vi "Dash_Hopper_Testing.vi"() -> ()   [LabVIEW 2017, in "Hopper System.lvlib"]
uses:
  Hopper System.lvlib
  Cluster_CMD to SM Data.ctl
  ENUM_Firing_State.ctl
  _SHARE ALL/Global Share All/Global_STOP.vi
  Globals/Global_CMD to SM Data.vi
  Global_Line-Fake.vi
  Global_SM_Data Out.vi
panel:
  in  "Line Sensor-Fake_Testor":bool
  in  "Hopper Stop_CMD":bool
  out "Hopper_SM_Loader Speed":dbl
  out "Hopper_SM_Center Speed":dbl
  in  "Inner Motor Speed":dbl=0.4
  in  "STOP":bool
  in  "Loader Speed":dbl=0.4
  in  "Hopper_CMD":T1={"Enable Loading"=FALSE, "Disable Loading"=FALSE, "Fireing State"=enum."No Fireing", "Time Limit Loading"=5.0, "Time Limit Rapid"=2.0, "Rapid Fire Shot Limit"=0, "Shotgun Fire Shot Limit"=0}
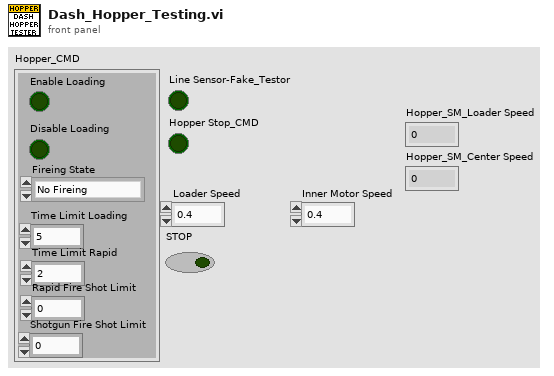
[diagram p1: front panel]
types:
  T1 = typedef "Hopper System.lvlib/Cluster_CMD to SM Data.ctl" = cluster{"Enable Loading":bool, "Disable Loading":bool, "Fireing State":T2, "Time Limit Loading":dbl, "Time Limit Rapid":dbl, "Rapid Fire Shot Limit":i32, "Shotgun Fire Shot Limit":i32}
  T2 = typedef "Hopper System.lvlib/ENUM_Firing_State.ctl" = enum16{"No Fireing", "Rapid Fire", "Shotgun Fireing"}
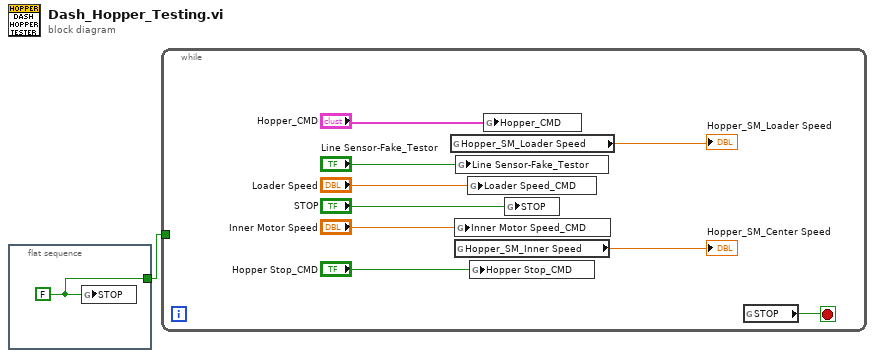
[diagram p0: block diagram]
diagram:
  n1 = flat-sequence {
    tunnel: [w2] -> w1
    frame #0 {
      w2 = FALSE ("STOP 2")
      n2 = global write "Global_STOP.vi" "STOP"(w2) -> ()
    }
  }
  n3 = while {
    tunnel: w1 -> [_]
    stop <- w9 stop-if-true
    n4 = global read "Global_SM_Data Out.vi" "Hopper_SM_Loader Speed"() -> (→"Hopper_SM_Loader Speed":dbl)
    n5 = global write "Global_CMD to SM Data.vi" "Inner Motor Speed_CMD"("Inner Motor Speed") -> ()
    n6 = global read "Global_SM_Data Out.vi" "Hopper_SM_Inner Speed"() -> (→"Hopper_SM_Center Speed":dbl)
    n7 = global write "Global_Line-Fake.vi" "Line Sensor-Fake_Testor"("Line Sensor-Fake_Testor") -> ()
    n8 = global write "Global_CMD to SM Data.vi" "Loader Speed_CMD"("Loader Speed") -> ()
    n9 = global write "Global_CMD to SM Data.vi" "Hopper Stop_CMD"("Hopper Stop_CMD") -> ()
    n10 = global write "Global_CMD to SM Data.vi" "Hopper_CMD"("Hopper_CMD") -> ()
    n11 = global write "Global_STOP.vi" "STOP"("STOP") -> ()
    n12 = global read "Global_STOP.vi" "STOP"() -> (w9:bool)
  }
